vi "shift_register.vi"() -> ()   [LabVIEW 2020]
panel:
  in  "stop":bool
  out "Dado dentro":dbl
  out "Dado fora":dbl
  in  "Incremento":dbl
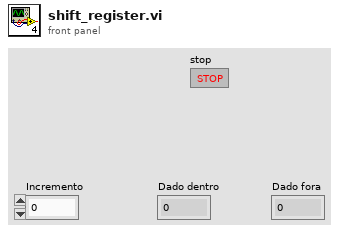
[diagram p1: front panel]
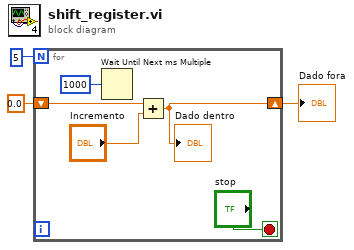
[diagram p0: block diagram]
diagram:
  n1 = for {
    N: 5 -> [_]
    shift-right: [w5] -> w2
    shift-left: 0.0 -> [w6]
    stop <- "stop" stop-if-true
    n2 = Wait Until Next ms Multiple(millisecond multiple=u32 1000) -> ()  [unwired: 1 out]
    n3 = Add(x=w6, y="Incremento") -> (x+y=w5:dbl)
    "Dado dentro" <- w5
  }
  "Dado fora" <- w2
